vi "Control select.vi"(7 "resousce name":string, 8 "error in (no error)":errorcluster, 11 "Clust Refnum":refnum<vi>) -> (0 "error out":errorcluster, 3 "Control Refnum":refnum<vi>)   [LabVIEW 2010]
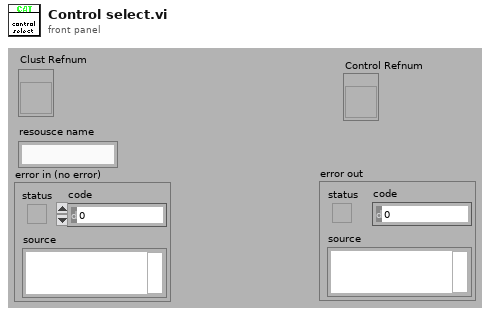
[diagram p1: front panel]
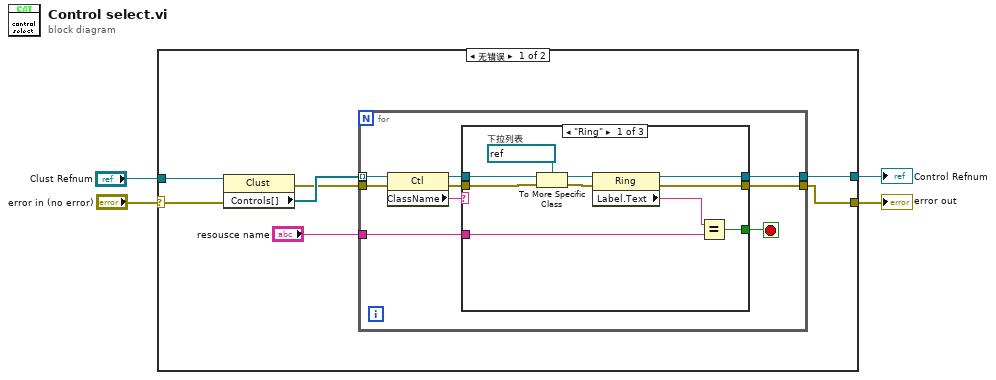
[diagram p0: block diagram]
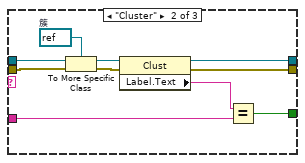
[diagram p2: hidden frame]
diagram:
  n1 = case shown="无错误" "error in (no error)" {
    selector: "error in (no error)" -> [w8 w42]
    tunnel: [w10 _] -> w4
    tunnel: [w9 w42] -> w3
    tunnel: "Clust Refnum" -> [w7 _]
    frame No Error {
      n2 = property class="Clust"(reference=w7, error in=w8) -> (error out=w5:errorcluster, "Controls[]"=w6:refnum<vi>[])  [unwired: 1 out]
      n3 = for {
        tunnel: w6 -> [w20] mode=indexing
        tunnel: w5 -> [w16]
        tunnel: "resousce name" -> [w15]
        tunnel: [w13] -> w10
        tunnel: [w12] -> w9
        stop <- w14 stop-if-true
        n4 = property class="Ctl"(reference=w20, error in=w16) -> (reference out=w18:refnum<vi>, error out=w17:errorcluster, "ClassName"=w19:string)
        n5 = case shown="\"Ring\"" w19 {
          tunnel: w18 -> [w29 w36 _]
          tunnel: w17 -> [w26 w35 w41]
          tunnel: w15 -> [w25 w31 _]
          tunnel: [w24 w32 _] -> w14
          tunnel: [w23 w34 _] -> w13
          tunnel: [w21 w33 w41] -> w12
          frame "Ring" {
            w30 = refnum<vi> refnum  # 下拉列表
            n6 = To More Specific Class(target class=w30, reference=w29, error in=w26) -> (specific class reference=w28:refnum<vi>, error out=w27:errorcluster)
            n7 = property class="Ring"(reference=w28, error in=w27) -> (reference out=w23:refnum<vi>, error out=w21:errorcluster, "Label.Text"=w22:string)
            n8 = Equal?(x=w22, y=w25) -> (x = y?=w24:bool)
          }
          frame "Cluster" {
            w40 = refnum<vi> refnum  # 簇
            n9 = To More Specific Class(target class=w40, reference=w36, error in=w35) -> (specific class reference=w39:refnum<vi>, error out=w38:errorcluster)
            n10 = property class="Clust"(reference=w39, error in=w38) -> (reference out=w34:refnum<vi>, error out=w33:errorcluster, "Label.Text"=w37:string)
            n11 = Equal?(x=w37, y=w31) -> (x = y?=w32:bool)
          }
          frame Default {
          }
        }
      }
    }
    frame Error {
    }
  }
  "Control Refnum" <- w4
  "error out" <- w3
